vi "UsesCents2DollarString.vi"() -> ()   [LabVIEW 2014]
panel:
  out "Dollar String Out":string
  in  "Numeric":dbl format="%#_13g"
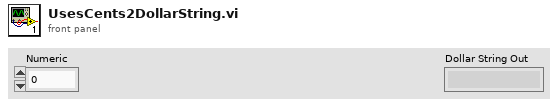
[diagram p1: front panel]
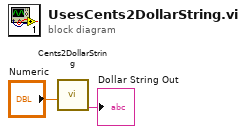
[diagram p0: block diagram]
diagram:
  n1 = call "Cents2DollarString.vi"("Numeric"="Numeric") -> ("Dollar String Out"=→"Dollar String Out":string)  [unwired: 10 in]
